vi "Pre Launch Init.vi"(11 "Devices to Load in":refnum<class "Devices to Load.lvclass">) -> (0 "error out":errorcluster, 3 "Devices to Load out":refnum<class "Devices to Load.lvclass">)   [LabVIEW 2018, in "Devices to Load Config Actor.lvlib" / "Devices to Load.lvclass"]
doc: "(<B>Filename</B>: Actor Framework.lvlib:Actor.lvclass:Pre Launch Init.vi)\n\nDefines behavior that occurs after the Launch Nested Actor method is invoked but before the actor's Actor Core method begins running.\n\nBy default, this method does nothing. A descendant class may override it to define behavior."
uses:
  Devices to Load.lvclass
  Controls/Devices to Load User Events.ctl
  Devices to Load.lvclass/Devices to Load.ctl
  <vilib>/ActorFramework/Actor/Actor.lvclass
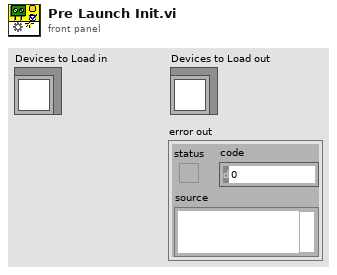
[diagram p1: front panel]
types:
  T1 = typedef "Devices to Load Config Actor.lvlib/Devices to Load.lvclass/Devices to Load User Events.ctl" = cluster{"ItemNames":refnum<user-event>, "stop":refnum<user-event>}
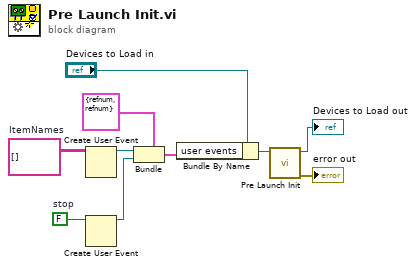
[diagram p0: block diagram]
diagram:
  w2 = FALSE  # stop
  w7 = string[][] []  # ItemNames
  n1 = Create User Event(user event datatype=w7) -> (user event=w5:refnum<user-event>)  [unwired: 1 in, 1 out]
  n2 = Create User Event(user event datatype=w2) -> (user event=w1:refnum<user-event>)  [unwired: 1 in, 1 out]
  n3 = Bundle(cluster=T1 {"ItemNames"=refnum, "stop"=refnum} ("user events"), "ItemNames"=w5, "stop"=w1) -> (w3:T1)
  n4 = Bundle By Name(cluster="Devices to Load in", "user events"=w3) -> (w4:refnum<class "Devices to Load.lvclass">)
  n5 = call-parent "Pre Launch Init.vi"("Actor in"=w4) -> ("error out"=→"error out":errorcluster, "Actor out"=→"Devices to Load out":refnum<class "Devices to Load.lvclass">)  [unwired: 9 in]
